vi "from string 1.0.vi"(8 "error in (no error)":errorcluster, 10 "data":string, 11 "Multiplexer configuration in":refnum<class "Multiplexer configuration.lvclass">) -> (0 "error out":errorcluster, 3 "Multiplexer configuration out":refnum<class "Multiplexer configuration.lvclass">)   [LabVIEW 2021, in "Multiplexer configuration.lvclass"]
uses:
  Multiplexer configuration.lvclass
  Multiplexer configuration.lvclass/Multiplexer configuration.ctl
  <vilib>/NI/Tag Bus Module Framework/channel/TBM channel.lvclass
  <vilib>/NI/Configuration Framework/serializable configuration/NISE_CEF_serializable configuration.lvclass
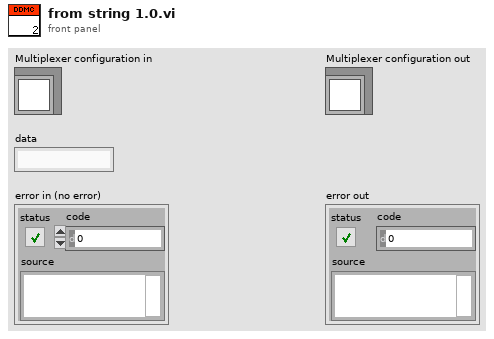
[diagram p1: front panel]
types:
  T1 = cluster{"[0]":refnum<class "TBM channel.lvclass">, "[1]":refnum<class "TBM channel.lvclass">, "[2]":refnum<class "TBM channel.lvclass">, "[3]":refnum<class "TBM channel.lvclass">}
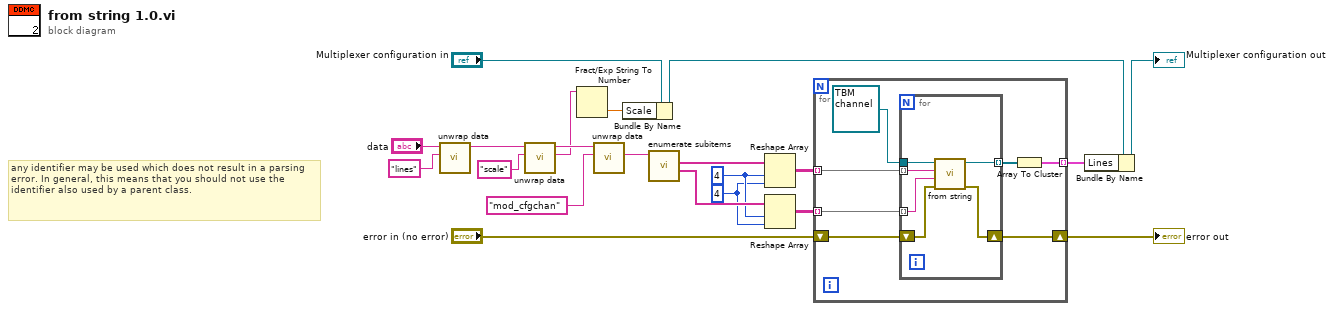
[diagram p0: block diagram]
diagram:
  w1 = 4 ("dimension size")
  w2 = 4 ("dimension size")
  # "any identifier may be used which does not result in a parsing error. In general, this means that you should not use the identifier also used by a parent class."
  n1 = call <vilib>:"unwrap data.vi"("identifier"="lines" ("additional identifier"), "data to unwrap"="data") -> ("remaining string"=w12:string)  [unwired: 8 in, 1 out]
  n2 = call <vilib>:"unwrap data.vi"("identifier"="scale", "data to unwrap"=w12) -> ("unwrapped data"=w9:string, "remaining string"=w11:string)  [unwired: 8 in]
  n3 = Fract/Exp String To Number(string=w9) -> (number=w7:dbl)  [unwired: 3 in, 1 out]
  n4 = call <vilib>:"unwrap data.vi"("identifier"="mod_cfgchan", "data to unwrap"=w11) -> ("unwrapped data"=w19:string)  [unwired: 8 in, 1 out]
  n5 = Bundle By Name(cluster="Multiplexer configuration in", "Scale"=w7) -> (w8:refnum<class "Multiplexer configuration.lvclass">)
  n6 = call <vilib>:"enumerate subitems.vi"("data to enumerate"=w19) -> ("associated data"=w3:string[], "discovered subitems"=w6:string[])  [unwired: 8 in, 1 out]
  n7 = Reshape Array(w6, w2, w1) -> (w5:string[][])
  n8 = Reshape Array(w3, w2, w1) -> (w4:string[][])
  n9 = for {
    shift-right: [w28] -> w21
    shift-left: "error in (no error)" -> [w27]
    tunnel: [w22] -> w20 mode=indexing
    tunnel: w5 -> [w25] mode=indexing
    tunnel: w4 -> [w24] mode=indexing
    n10 = for {
      tunnel: refnum<class "TBM channel.lvclass"> refnum ("channel in") -> [w32]
      shift-right: [w34] -> w28
      shift-left: w27 -> [w33]
      tunnel: w25 -> [w31] mode=indexing
      tunnel: w24 -> [w30] mode=indexing
      tunnel: [w29] -> w23 mode=indexing
      n11 = call-dynamic "from string.vi"("error in"=w33, "channel data"=w30, "identifier"=w31, "channel in"=w32) -> ("error out"=w34:errorcluster, "channel out"=w29:refnum<class "TBM channel.lvclass">)  [unwired: 6 in]
    }
    n12 = Array To Cluster(array=w23) -> (cluster=w22:T1)
  }
  "error out" <- w21
  n13 = Bundle By Name(cluster=w8, "Lines"=w20) -> (→"Multiplexer configuration out":refnum<class "Multiplexer configuration.lvclass">)
